vi "setGain.vi"(8 "error in (no error)":errorcluster, 10 "Gain":dbl, 11 "OptCtrl in":refnum<class "OptCtrl.lvclass">) -> (0 "error out":errorcluster, 3 "OptCtrl out":refnum<class "OptCtrl.lvclass">)   [LabVIEW 2016, in "OptCtrl.lvclass"]
uses:
  OptCtrl.lvclass
  OptCtrl.lvclass/OptCtrl.ctl
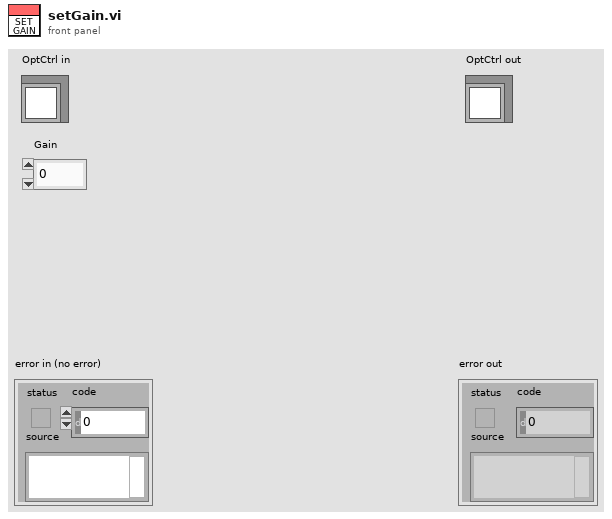
[diagram p1: front panel]
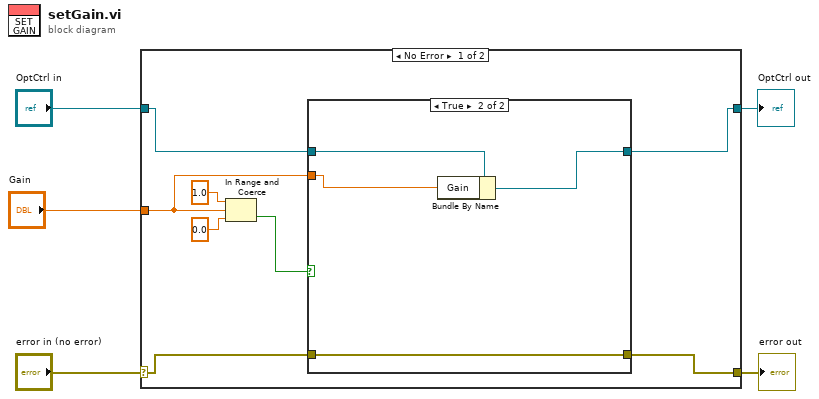
[diagram p0: block diagram]
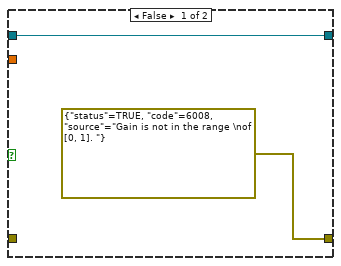
[diagram p2: hidden frame]
diagram:
  n1 = case shown="No Error" "error in (no error)" {
    selector: "error in (no error)" -> [w9 w21]
    tunnel: [w10 w21] -> w4
    tunnel: [w8 w20] -> w1
    tunnel: "OptCtrl in" -> [w7 w20]
    tunnel: "Gain" -> [w6 _]
    frame No Error {
      n2 = In Range and Coerce(upper limit=1.0, x=w6, lower limit=0.0) -> (In Range?=w11:bool)  [unwired: 1 out]
      n3 = case shown="True" w11 {
        tunnel: [errorcluster {"status"=TRUE, "code"=6008, "source"="Gain is not in the range \nof [0, 1]. "} ("error IO") w19] -> w10
        tunnel: w9 -> [_ w19]
        tunnel: [w14 w17] -> w8
        tunnel: w7 -> [w14 w18]
        tunnel: w6 -> [_ w16]
        frame False {
        }
        frame True {
          n4 = Bundle By Name(cluster=w18, "Gain"=w16) -> (w17:refnum<class "OptCtrl.lvclass">)
        }
      }
    }
    frame Error {
    }
  }
  "error out" <- w4
  "OptCtrl out" <- w1
